vi "Enqueue XYZ.vi"(0 "X":dbl, 1 "Y":dbl, 2 "Z":dbl, 3 "X Has Value?":bool, 4 "Y Has Value?":bool, 5 "Z Has Value?":bool) -> ()   [LabVIEW 2011]
uses:
  point.ctl
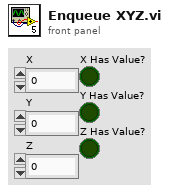
[diagram p1: front panel]
types:
  T1 = typedef "point.ctl" = cluster{"X":dbl, "Y":dbl, "Z":dbl, "Ramp":dbl, "Speed":dbl}
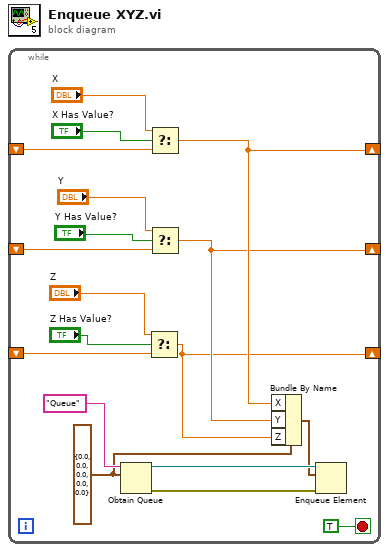
[diagram p0: block diagram]
diagram:
  n1 = while {
    shift-right: [w5] -> _
    shift-left: _ -> [w16]
    shift-right: [w4] -> _
    shift-left: _ -> [w13]
    shift-right: [w3] -> _
    shift-left: _ -> [w11]
    stop <- TRUE stop-if-true
    w6 = T1 {"X"=0.0, "Y"=0.0, "Z"=0.0, "Ramp"=0.0, "Speed"=0.0} ("Point")
    n2 = Obtain Queue(name (unnamed)="Queue", element data type=w6) -> (queue out=w8:refnum<queue>, error out=w7:errorcluster)  [unwired: 3 in, 1 out]
    n3 = Select(t="Z", s="Z Has Value?", f=w11) -> (s? t:f=w3:dbl)
    n4 = Select(t="X", s="X Has Value?", f=w16) -> (s? t:f=w5:dbl)
    n5 = Select(t="Y", s="Y Has Value?", f=w13) -> (s? t:f=w4:dbl)
    n6 = Bundle By Name(cluster=w6, "X"=w5, "Y"=w4, "Z"=w3) -> (w2:T1)
    n7 = Enqueue Element(queue=w8, element=w2, error in (no error)=w7) -> ()  [unwired: 1 in, 3 out]
  }
